vi "editDialog.vi"(0 "reference":refnum<class "AbstractNode.lvclass">, 1 "insidePackageNode":bool, 5 "error in (no error)":errorcluster) -> (14 "reference out":refnum<class "AbstractNode.lvclass">, 15 "changeConnection":T1, 16 "cancel":bool, 19 "error out":errorcluster)   [LabVIEW 2014, in "AbstractNode.lvclass"]
doc: "Edit Dialog"
uses:
  <resource>/Framework/Providers/Open_GDS/UML/AbstractNode_class/AbstractNode.lvclass
  <resource>/Framework/Providers/Open_GDS/UML/AbstractNode_class/private/NodeConnectionStatsType.ctl
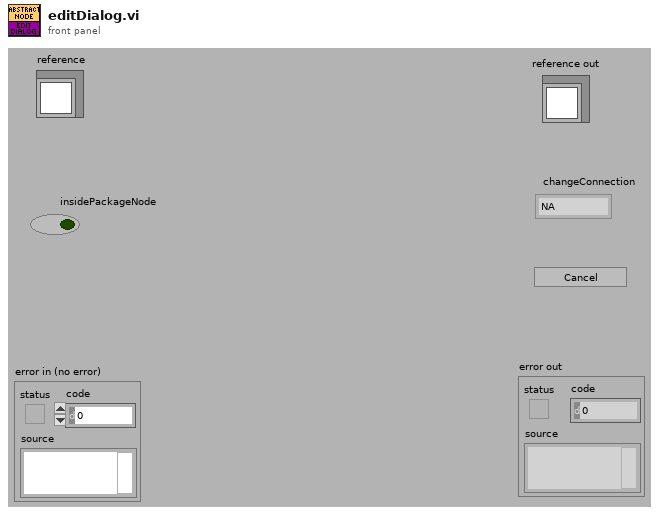
[diagram p1: front panel]
types:
  T1 = typedef "AbstractNode.lvclass/NodeConnectionStatsType.ctl" = enum16{"NA", "Connect", "DisConnect"}
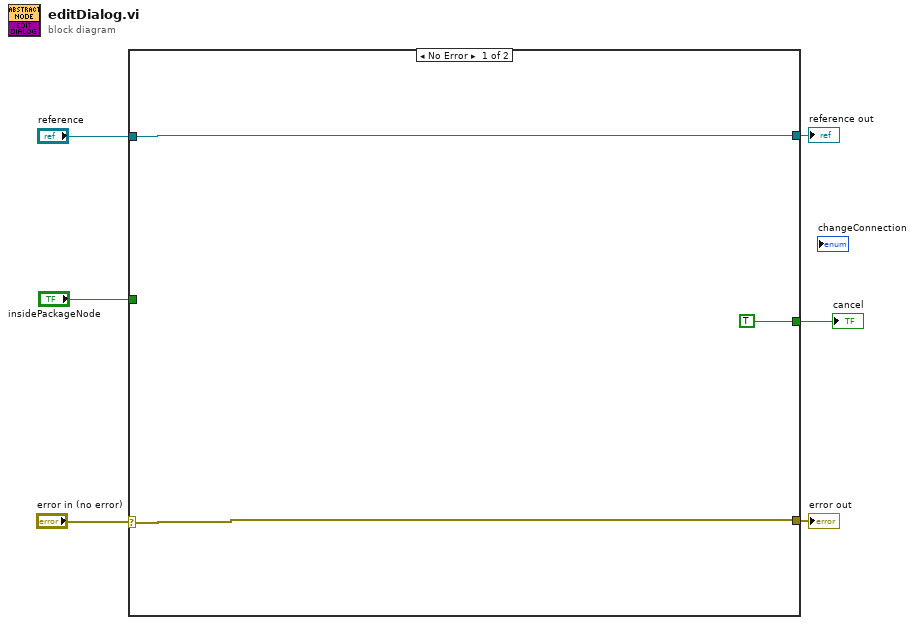
[diagram p0: block diagram]
diagram:
  n1 = case shown="No Error" "error in (no error)" {
    selector: "error in (no error)" -> [w8 w10]
    tunnel: "reference" -> [w9 w11]
    tunnel: [w8 w10] -> w5
    tunnel: [w9 w11] -> w4
    tunnel: "insidePackageNode" -> [_ _]
    tunnel: [TRUE ("cancel") _] -> w1
    frame No Error {
    }
    frame Error {
    }
  }
  "reference out" <- w4
  "error out" <- w5
  "cancel" <- w1
